vi "接收过程处理.vi"(6 "接收数据量":u32, 9 "reference输入":refnum<vi>, 10 "Str引用句柄":refnum<vi>, 11 "String输入":refnum<vi>) -> ()   [LabVIEW 2016]
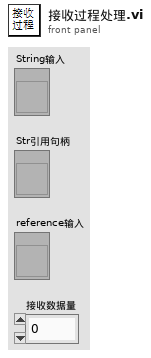
[diagram p1: front panel]
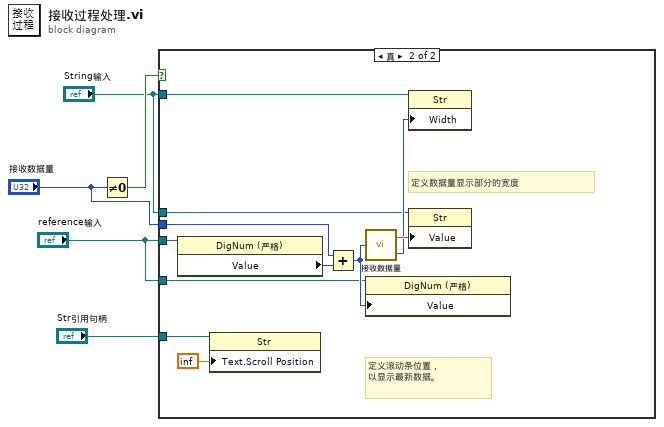
[diagram p0: block diagram]
diagram:
  n1 = Not Equal To 0?(x="接收数据量") -> (x != 0?=w4:bool)
  n2 = case shown="真" w4 {
    tunnel: "接收数据量" -> [_ w7]
    tunnel: "String输入" -> [_ w12]
    tunnel: "String输入" -> [_ w11]
    tunnel: "Str引用句柄" -> [_ w10]
    tunnel: "reference输入" -> [_ w9]
    tunnel: "reference输入" -> [_ w8]
    frame False {
    }
    frame True {
      # "定义滚动条位置，\n以显示最新数据。"
      # "定义数据量显示部分的宽度"
      n3 = property class="DigNum (严格)"(reference=w9) -> ("Value"=w14:u32)  [unwired: 1 in, 2 out]
      n4 = property on="属性节点" class="Str"(reference=w10, "Text.Scroll Position"=inf) -> ()  [unwired: 1 in, 2 out]
      n5 = Add(x=w7, y=w14) -> (x+y=w13:u32)
      n6 = call "接收数据量.vi"("数值"=w13) -> ("字符串"=w16:string, "x*y"=w15:i32)
      n7 = property class="DigNum (严格)"(reference=w8, "Value"=w13) -> ()  [unwired: 1 in, 2 out]
      n8 = property on="属性节点" class="Str"(reference=w11, "Width"=w15) -> ()  [unwired: 1 in, 2 out]
      n9 = property class="Str"(reference=w12, "Value"=w16) -> ()  [unwired: 1 in, 2 out]
    }
  }
